vi "Destroy.vi"(8 "Error In":errorcluster, 11 "reference in":refnum<class "Instrument.lvclass">) -> (0 "Error Out":errorcluster, 3 "reference out":refnum<class "Instrument.lvclass">)   [LabVIEW 2023, in "HAL GOOP4.lvlib" / "Instrument.lvclass"]
uses:
  Instrument.lvclass
  Interfaces/IConfigure/IConfigure.lvclass
  Instrument.lvclass/Instrument.ctl
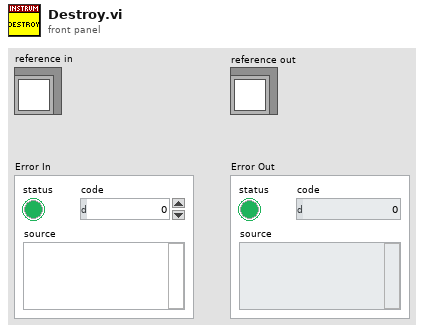
[diagram p1: front panel]
types:
  T1 = typedef "HAL GOOP4.lvlib/Instrument.lvclass/ObjectAttributes.ctl" = cluster{"IConfigure":refnum<class "IConfigure.lvclass">, "Ref Count":i16, "Start Count":i16}
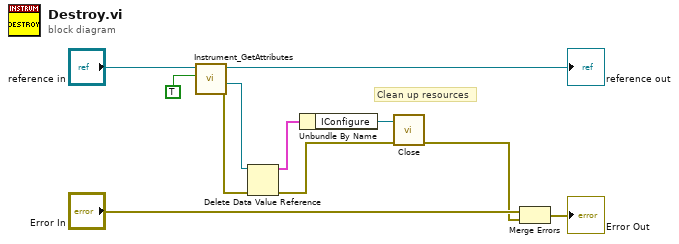
[diagram p0: block diagram]
diagram:
  # "Clean up resources"
  n1 = call "Instrument_GetAttributes.vi"("OnlyGetDvrReference(False)"=TRUE, "reference in"="reference in") -> ("Error Out"=w8:errorcluster, "DataRef"=w7:refnum<data-value>, "reference out"=→"reference out":refnum<class "Instrument.lvclass">)  [unwired: 6 in, 1 out]
  n2 = Delete Data Value Reference(data value reference=w7, error in=w8) -> (data value=w4:T1, error out=w2:errorcluster)
  n3 = Unbundle By Name(w4) -> ("IConfigure"=w3:refnum<class "IConfigure.lvclass">)
  n4 = call-dynamic "Close.vi"("error in (no error)"=w2, "IConfigure in"=w3) -> ("error out"=w1:errorcluster)  [unwired: 8 in, 1 out]
  n5 = Merge Errors("Error In", w1) -> (→"Error Out":errorcluster)
